vi "ExecuteAction.vi"(8 "error in (no error)":errorcluster, 10 "ButtonDefinition":T1) -> (0 "error out":errorcluster)   [LabVIEW 2021]
uses:
  VerticalButtonBar/ButtonCollection/ButtonDefinition.ctl
  .Externals/ButtonAction/ButtonAction.lvclass
  e2e359f8-865c-46d2-be85-a7a6c724827c.vi
  <vilib>/TriekselSoft/TracerLibrary/TracerLibrary/Tracer/protected/SendMessage.vi
  <vilib>/TriekselSoft/TracerLibrary/TracerLibrary/Tracer/protected/Timestamp.vi
  e2e359f8-865c-46d2-be85-a7a6c724827c.vi/f75db090-0877-4668-94fb-75c2140b1617.vi
  <vilib>/TriekselSoft/TracerLibrary/TracerLibrary/Tracer/Tracer_Level-Info.vi
  <vilib>/JDP Science/JSONtext/Variant to JSON Text.vi
  <vilib>/TriekselSoft/TracerLibrary/TracerLibrary/Tracer/protected/Tracer_ClassAttributes.vi
  <vilib>/JDP Science/JSONtext/LVClass Serializer/JSONtext LVClass Serializer.lvclass
  TemplateGUI.lvclass/TemplateGUI.ctl
  .Externals/Library_TSFramework_ApplicationArchitecture/Application/Application.lvclass
  VerticalButtonBar/ButtonCollection/ButtonCollection.lvclass
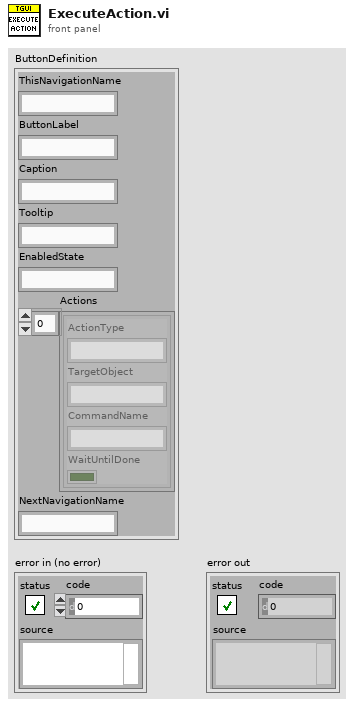
[diagram p1: front panel]
types:
  T1 = typedef "ButtonCollection.lvclass/ButtonDefinition.ctl" = cluster{"ThisNavigationName":string, "ButtonLabel":string, "Caption":string, "Tooltip":string, "EnabledState":string, "Actions":cluster{"ActionType":string, "TargetObject":string, "CommandName":string, "WaitUntilDone":bool}[], "NextNavigationName":string}
  T2 = cluster{"ActionType":string, "TargetObject":string, "CommandName":string, "WaitUntilDone":bool}[]
  T3 = cluster{"ButtonLabel":string, "Caption":string, "Cluster":cluster{"ActionType":string, "TargetObject":string, "CommandName":string, "WaitUntilDone":bool}}
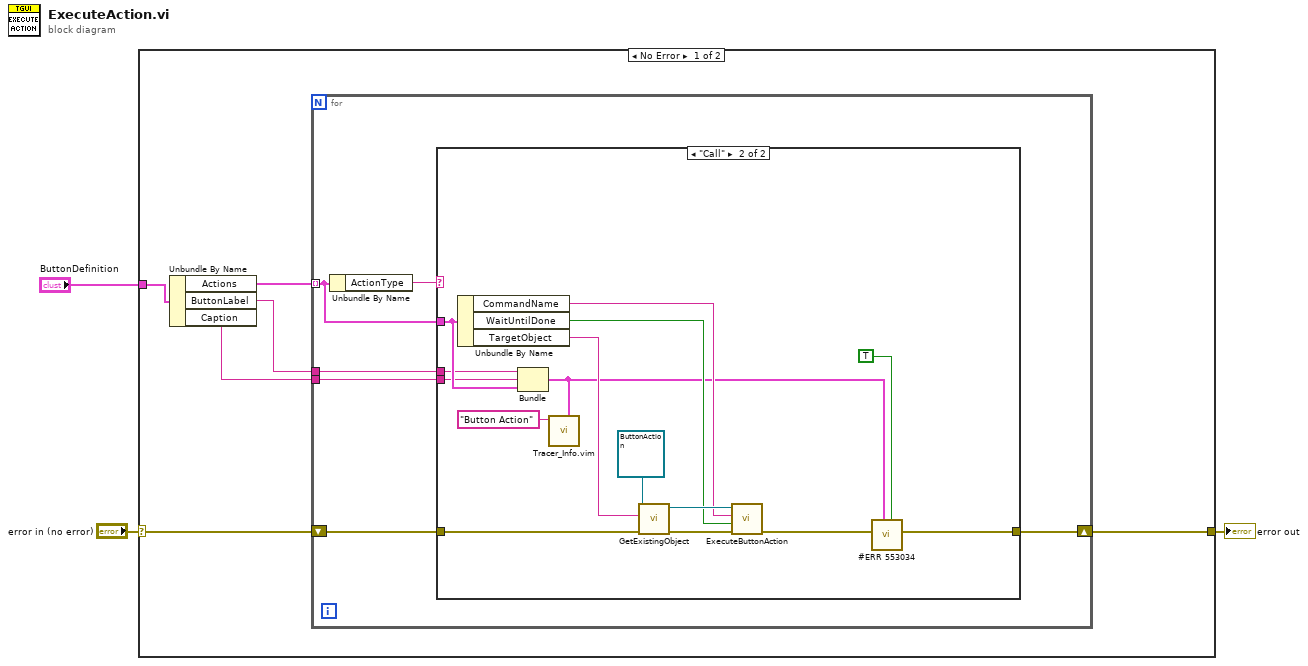
[diagram p0: block diagram]
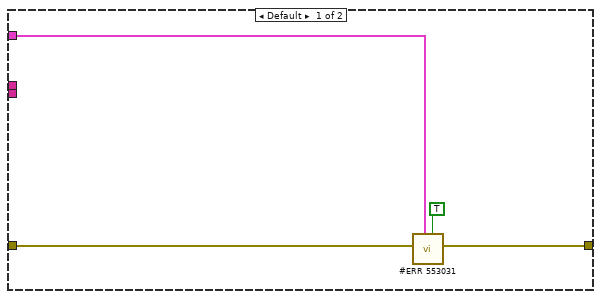
[diagram p2: hidden frame]
diagram:
  n1 = case shown="No Error" "error in (no error)" {
    selector: "error in (no error)" -> [w7 w35]
    tunnel: [w6 w35] -> w2
    tunnel: "ButtonDefinition" -> [w9 _]
    frame No Error {
      n2 = Unbundle By Name(w9) -> ("Actions"=w8:T2, "ButtonLabel"=w4:string, "Caption"=w5:string)
      n3 = for {
        tunnel: w8 -> [w12] mode=indexing
        shift-right: [w13] -> w6
        shift-left: w7 -> [w14]
        tunnel: w5 -> [w11]
        tunnel: w4 -> [w10]
        n4 = Unbundle By Name(w12) -> ("ActionType"=w15:string)
        n5 = case shown="\"Call\"" w15 {
          tunnel: [w18 w22] -> w13
          tunnel: w14 -> [w19 w34]
          tunnel: w12 -> [w17 w25]
          tunnel: w11 -> [_ w24]
          tunnel: w10 -> [_ w23]
          frame Default {
            n6 = call "#ERR 553031"("MergeErrors"=TRUE, "Data"=w17, "error in (no error)"=w19) -> ("error out"=w18:errorcluster)  [unwired: 8 in]
          }
          frame "Call" {
            n7 = Unbundle By Name(w25) -> ("CommandName"=w27:string, "WaitUntilDone"=w28:bool, "TargetObject"=w33:string)
            n8 = Bundle("ButtonLabel"=w23, "Caption"=w24, "Cluster"=w25) -> (w21:T3)  [unwired: 1 in]
            n9 = call "Tracer_Info.vim"("Data"=w21, "InfoText"="Button Action") -> ()  [unwired: 9 in, 1 out]
            n10 = call "GetExistingObject.vi"("error in (no error)"=w34, "ObjectName"=w33, "Type"=refnum<class "ButtonAction.lvclass"> refnum ("ButtonAction")) -> ("error out"=w31:errorcluster, "ObjectOut"=w29:refnum<class "ButtonAction.lvclass">)  [unwired: 7 in]
            n11 = call-dynamic "ExecuteButtonAction.vi"("Error In"=w31, "WaitForReply"=w28, "Command"=w27, "object in"=w29) -> ("Error Out"=w30:errorcluster)  [unwired: 6 in, 1 out]
            n12 = call "#ERR 553034"("MergeErrors"=TRUE, "Data"=w21, "error in (no error)"=w30) -> ("error out"=w22:errorcluster)  [unwired: 8 in]
          }
        }
      }
    }
    frame Error {
    }
  }
  "error out" <- w2
